vi "TEMP--Read Image on Button.vi"(9 "image item":i32, 11 "File with Button":path) -> (0 "error out":errorcluster, 3 "png file out":path)   [LabVIEW 2021]
doc: "This example VI was obtained from this post. This strips out the saving profile and just reads the image on an existing button.\n\nhttps://forums.ni.com/t5/LabVIEW-APIs-Discussions/Set-TRUE-FALSE-Image-of-a-boolean-control-automatically-using/m-p/3419083/highlight/true#M868\n\n<b>WARNING</b>\nThis VI uses a dll call to the resource file for a LabVIEW VI/CTL - it is searching the binary data for the PNG images that the VI or CTL contains\n\n<b>Code Developed By:</b>\nTechnology Service Corporation\n1983 S Liberty Drive\nBloomington, IN 47403\nPhone: 812 558-7100\nwww.tsc.com/atcs\n\nDeveloper:\nDaniel Coons"
uses:
  <vilib>/Utility/traverseref.llb/TRef TravTarget.ctl
  <vilib>/Utility/traverseref.llb/VI Scripting - Traverse.lvlib
panel:
  out "size(s)":i32
  out "Array 4":i32[](array[numeric])
  out "Array 3":string[](array[string])
  out "Array 2":i32[](array[numeric])
  out "Array":i32[](array[numeric])
  out "resources":T1(array[cluster])
  out "Resources":string[](array[string])
  # "MNGI resources are 6 images\non buttons (pressed, hover, etc)\n\n-When set to a \"decal\", it should\nbe the only one"
  # "For DEBUG"
  # "tonal--icons--rounded"
  # "4"
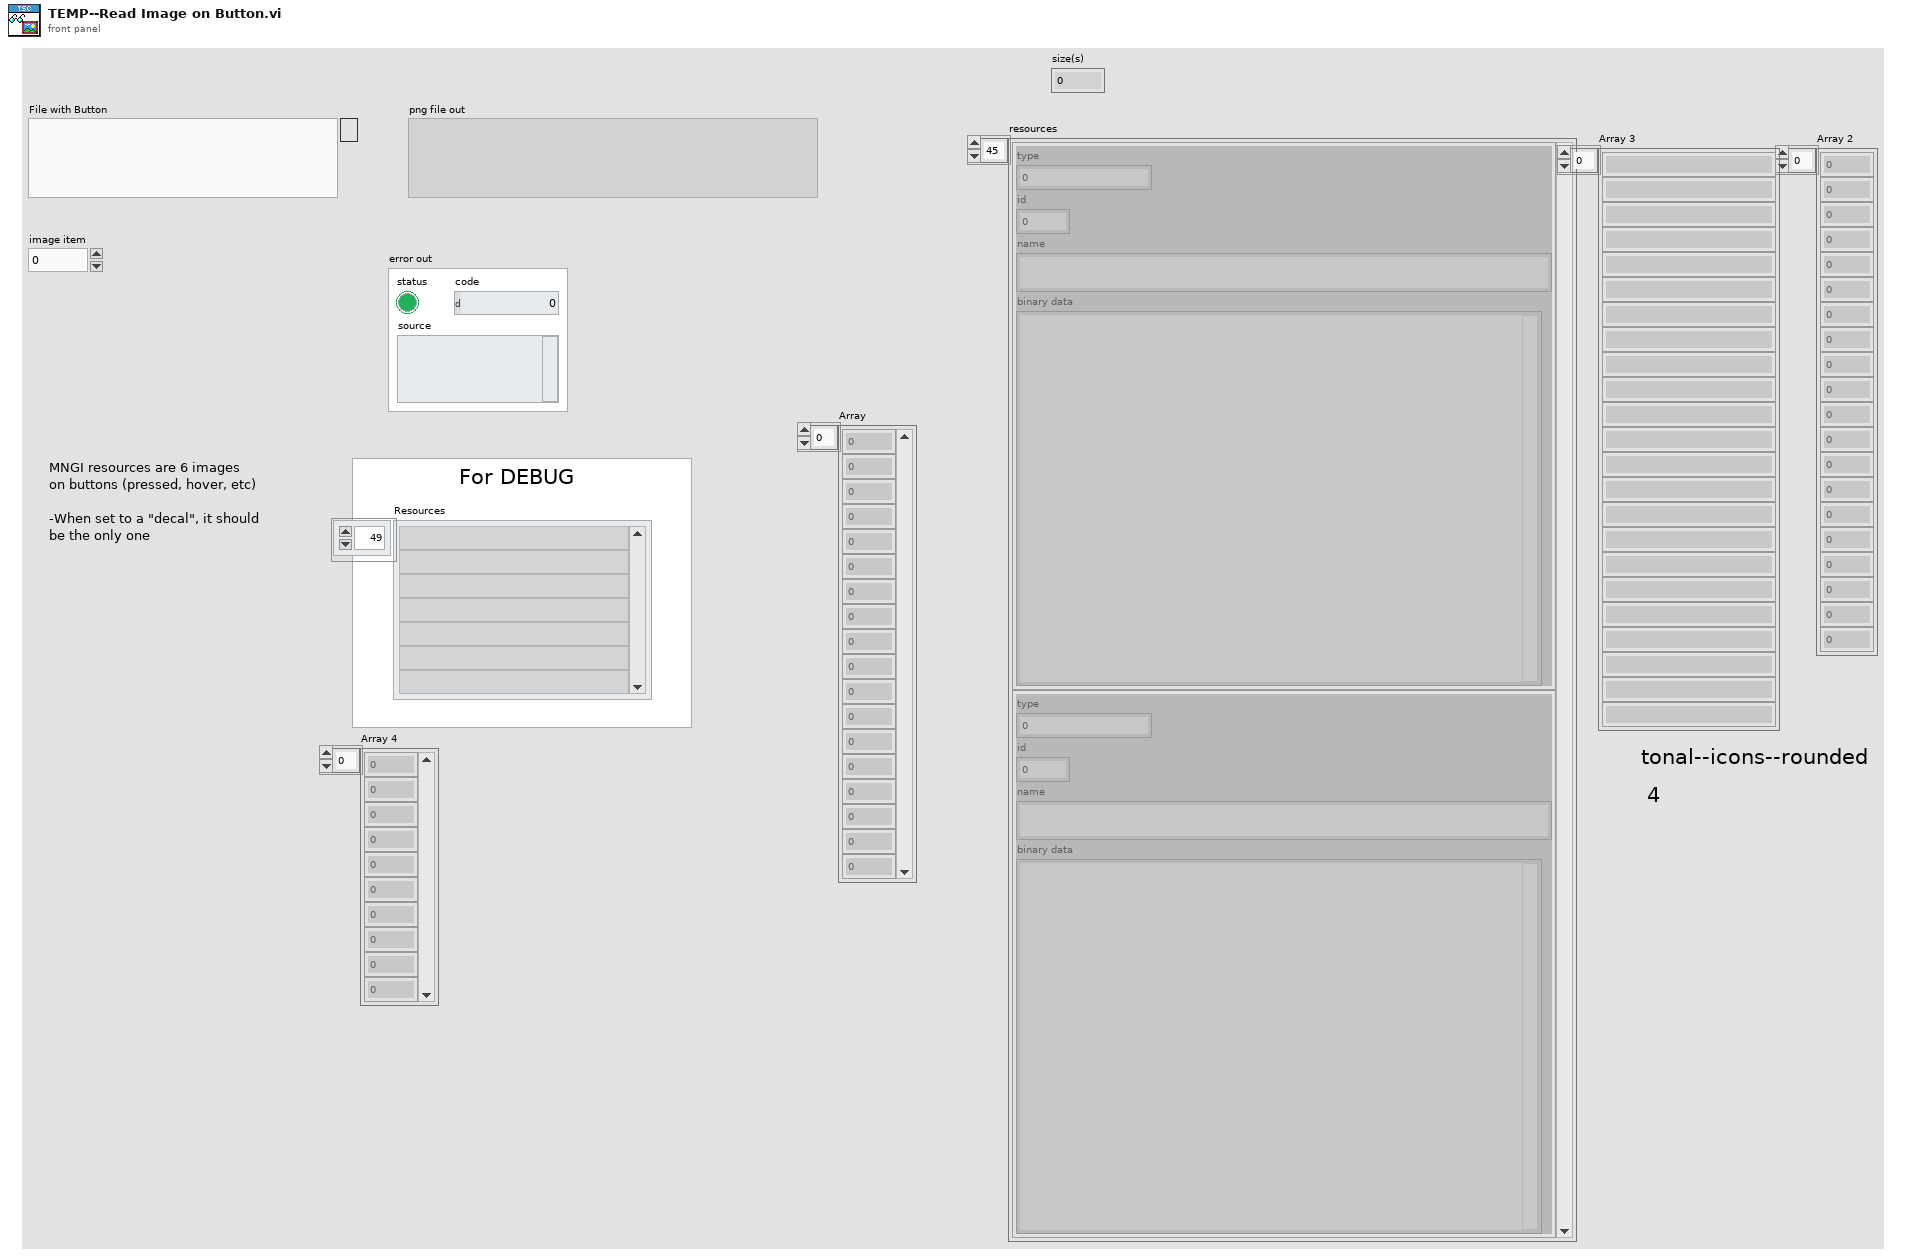
[diagram p1: front panel]
types:
  T1 = cluster{"type":u32, "id":i32, "name":string, "binary data":string}[]
  T2 = enum16{"open", "replace", "create", "open or create", "replace or create", "replace or create with confirmation"}
  T3 = typedef "TRef TravTarget.ctl" = enum16{"FP", "BD", "Other"}
  T4 = cluster{"type":u32, "id":i32, "name":string, "binary data":string}
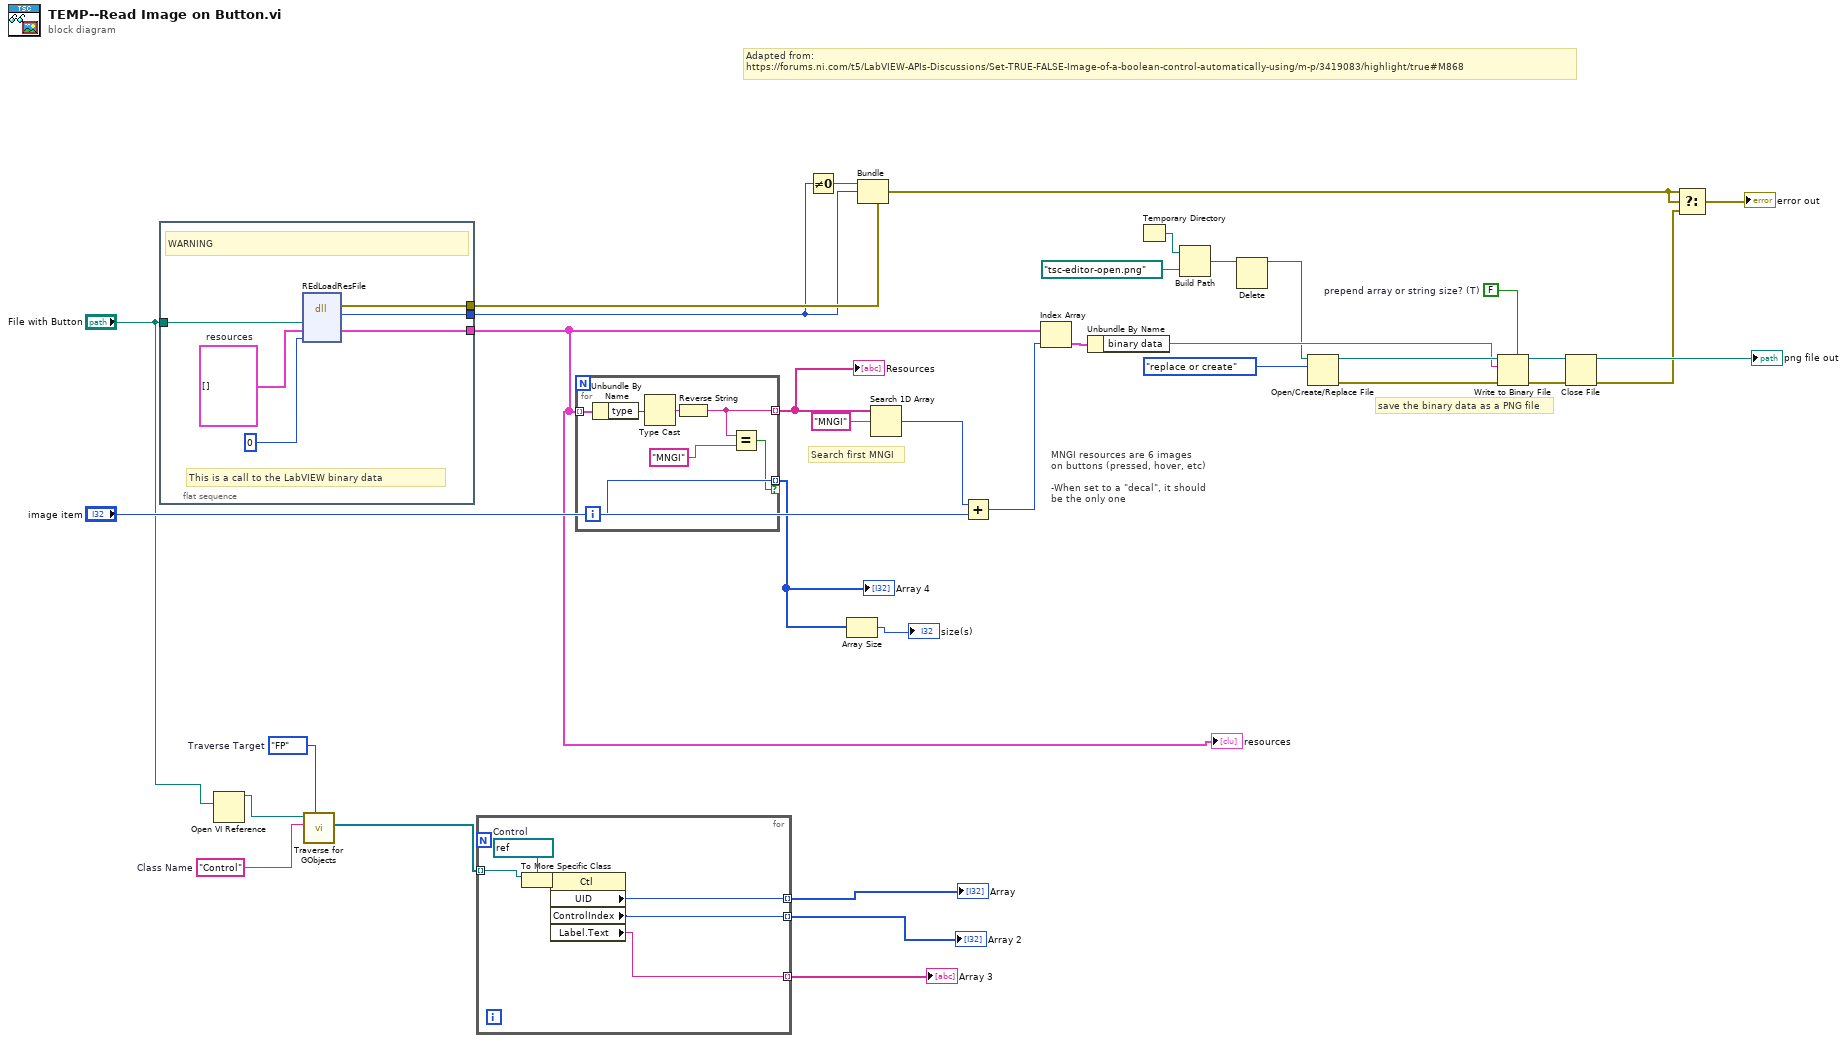
[diagram p0: block diagram]
diagram:
  w3 = FALSE  # prepend array or string size? (T)
  w20 = TRef_TravTarget."FP"  # Traverse Target
  w21 = "Control"  # Class Name
  # "save the binary data as a PNG file"
  # "MNGI resources are 6 images\non buttons (pressed, hover, etc)\n\n-When set to a \"decal\", it should\nbe the only one"
  # "Adapted from:\nhttps://forums.ni.com/t5/LabVIEW-APIs-Discussions/Set-TRUE-FALSE-Image-of-a-boolean-control-automatically-using/m-p/3419083/highlight/true#M868"
  # "Search first MNGI"
  n1 = flat-sequence {
    tunnel: [w39] -> w35
    tunnel: [w38] -> w33
    tunnel: "File with Button" -> [w37]
    tunnel: [w36] -> w24
    frame #0 {
      w41 = T1 []  # resources
      # "This is a call to the LabVIEW binary data"
      # "WARNING"
      n2 = dll-call lib="LabVIEW" fn="REdLoadResFile"("path"=w37, "resources"=w41, "type"=0) -> (error out=w39:errorcluster, "return type"=w38:i32, "resources"=w36:T1)  [unwired: 3 in, 3 out]
    }
  }
  n3 = Open VI Reference(vi path="File with Button") -> (vi reference=w22:refnum<vi>)  [unwired: 5 in, 1 out]
  n4 = call <vilib>:"Traverse for GObjects.vi"("Traverse Target"=w20, "Class Name"=w21, "VI Refnum"=w22) -> ("References"=w19:refnum<vi>[])  [unwired: 5 in, 3 out]
  n5 = for {
    tunnel: w19 -> [w47] mode=indexing
    tunnel: [w46] -> w18 mode=indexing
    tunnel: [w43] -> w17 mode=indexing
    tunnel: [w42] -> w16 mode=indexing
    w44 = refnum<vi> refnum  # Control
    n6 = To More Specific Class(target class=w44, reference=w47) -> (specific class reference=w45:refnum<vi>)  [unwired: 1 in, 1 out]
    n7 = property class="Ctl"(reference=w45) -> ("UID"=w46:i32, "ControlIndex"=w43:i32, "Label.Text"=w42:string)  [unwired: 1 in, 2 out]
  }
  "Array" <- w18
  "Array 2" <- w17
  "Array 3" <- w16
  n8 = for {
    tunnel: w24 -> [w54] mode=indexing
    tunnel: [w50] -> w25 mode=indexing
    tunnel: [w49] -> w2 mode=indexing if=w48
    i -> [w49]
    n9 = Unbundle By Name(w54) -> ("type"=w52:u32)
    n10 = Type Cast(x=w52) -> (*(type *) &x=w53:string)  [unwired: 1 out]
    n11 = Reverse String(1:w53) -> (0:w50:string)
    n12 = Equal?(x=w50, y="MNGI" ("element")) -> (x = y?=w48:bool)
  }
  "Resources" <- w25
  "Array 4" <- w2
  n13 = Not Equal To 0?(x=w33) -> (x != 0?=w34:bool)
  n14 = Array Size(array=w2) -> (size(s)=→"size(s)":i32)
  n15 = Bundle(cluster=w35, "status"=w34, "code"=w33) -> (w31:errorcluster)  [unwired: 1 out]
  n16 = Search 1D Array(1D array=w25, element="MNGI") -> (index of element=w28:i32)  [unwired: 1 out]
  n17 = Add(x=w28, y="image item") -> (x+y=w29:i32)
  n18 = Index Array(array=w24, index=w29) -> (element=w15:T4)
  n19 = Unbundle By Name(w15) -> ("binary data"=w8:string)
  n20 = Temporary Directory() -> (w14:path)
  n21 = Build Path(base path=w14, name or relative path=path "tsc-editor-open.png") -> (appended path=w12:path)
  n22 = Delete(path (use dialog)=w12) -> (deleted path=w4:path)  [unwired: 4 in, 2 out]
  n23 = Open/Create/Replace File(file path (use dialog)=w4, operation (0:open)=T2."replace or create") -> (refnum out=w9:refnum<file>, error out=w10:errorcluster)  [unwired: 4 in, 1 out]
  n24 = Write to Binary File(file (use dialog)=w9, data=w8, error in=w10, 5:w3) -> (refnum out=w6:refnum<file>, error out=w7:errorcluster)  [unwired: 2 in, 1 out]
  n25 = Close File(refnum=w6, error in=w7) -> (path=→"png file out":path, error out=w5:errorcluster)
  n26 = Select(t=w31, s=w31, f=w5) -> (s? t:f=→"error out":errorcluster)
  "resources" <- w24
